vi "Key Split.vi"(11 "Key":string) -> (3 "Key Elements":string[](array[string]))   [LabVIEW 2023]
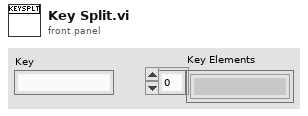
[diagram p1: front panel]
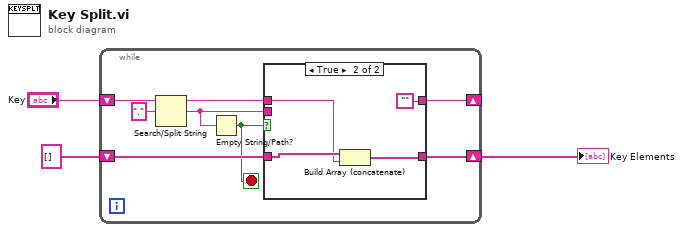
[diagram p0: block diagram]
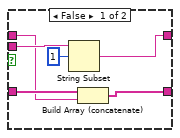
[diagram p2: hidden frame]
diagram:
  n1 = while {
    shift-right: [w5] -> _
    shift-left: "Key" -> [w11]
    shift-right: [w8] -> w1
    shift-left: string[] [] -> [w9]
    stop <- w7 stop-if-true
    n2 = Search/Split String(string=w11, search string/char (-)=".") -> (substring before match=w4:string, match + rest of string=w6:string)  [unwired: 1 in, 1 out]
    n3 = Empty String/Path?(string/path=w6) -> (empty?=w7:bool)
    n4 = case shown="True" w7 {
      tunnel: w9 -> [w14 w20]
      tunnel: [w12 w18] -> w8
      tunnel: w6 -> [w17 _]
      tunnel: [w16 ""] -> w5
      tunnel: w4 -> [w13 w19]
      frame False {
        n5 = String Subset(string=w17, offset (0)=1) -> (substring=w16:string)  [unwired: 1 in]
        n6 = Build Array (concatenate)(w14, w13) -> (w12:string[])
      }
      frame True {
        n7 = Build Array (concatenate)(w20, w19) -> (w18:string[])
      }
    }
  }
  "Key Elements" <- w1
